vi "综合生物毒性电源命令.vi"(10 "通电/断电":bool, 11 "队列":refnum<queue>) -> (3 "队列输出":refnum<queue>)   [LabVIEW 2016, in "PLC.lvlib"]
uses:
  PLC.lvlib
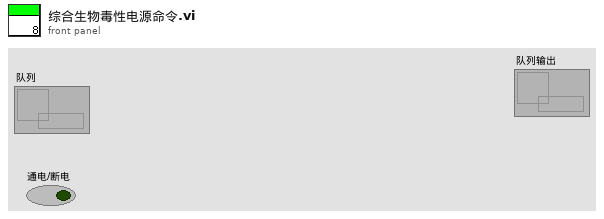
[diagram p1: front panel]
types:
  T1 = typedef "采配水类型.ctl" = enum16{"V1", "V2", "V3", "V4", "室内V1", "室内V2", "固定站V1", "固定站V2", "浮船V1", "浮船V2", "养殖尾水", "广东华南所"}
  T2 = cluster{"命令":string, "数据":cluster{"starting address":u16, "holding register value":u16}}
  T3 = cluster{"命令":string, "data":cluster{"starting address":u16, "coil values":bool[]}}
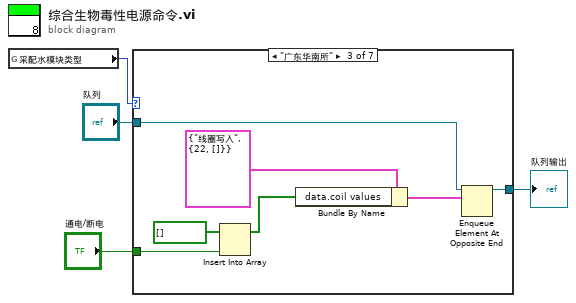
[diagram p0: block diagram]
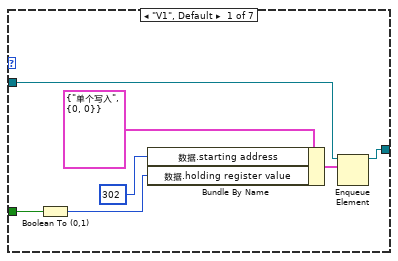
[diagram p2: hidden frame]
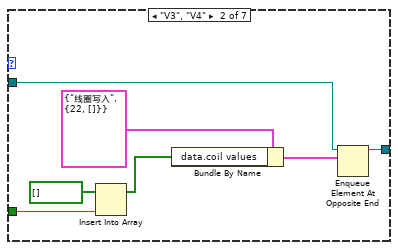
[diagram p3: hidden frame]
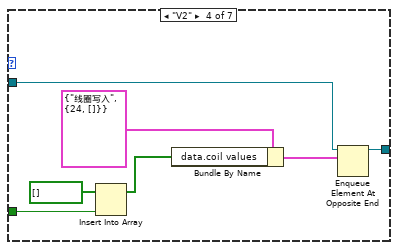
[diagram p4: hidden frame]
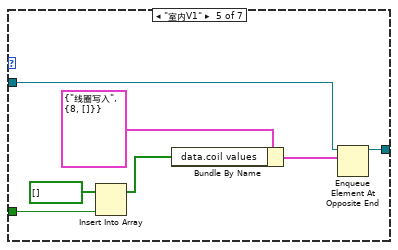
[diagram p5: hidden frame]
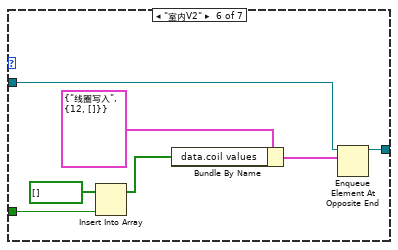
[diagram p6: hidden frame]
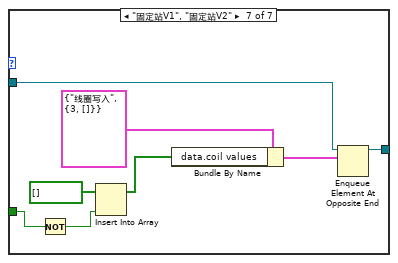
[diagram p7: hidden frame]
diagram:
  n1 = global read "系统设置全局变量.vi" "采配水模块类型"() -> (w1:T1)
  n2 = case shown="\"广东华南所\"" w1 {
    tunnel: "队列" -> [w9 w17 w24 w31 w38 w45 w53]
    tunnel: [w8 w16 w23 w30 w37 w44 w52] -> w3
    tunnel: "通电/断电" -> [w6 w15 w22 w29 w36 w43 w51]
    frame "V1", Default {
      n3 = Boolean To (0,1)(Boolean=w6) -> (0, 1=w5:i16)
      n4 = Bundle By Name(cluster=T2 {"命令"="单个写入", "数据"={"starting address"=0, "holding register value"=0}} ("元素"), "数据.starting address"=u16 302, "数据.holding register value"=w5) -> (w7:T2)
      n5 = Enqueue Element(queue=w9, element=w7) -> (queue out=w8:refnum<queue>)  [unwired: 2 in, 2 out]
    }
    frame "V3", "V4" {
      n6 = Insert Into Array(array=bool[] [] ("data.coil values"), new element=w15) -> (w12:bool[])  [unwired: 1 in]
      n7 = Bundle By Name(cluster=T3 {"命令"="线圈写入", "data"={"starting address"=22, "coil values"=[]}} ("元素"), "data.coil values"=w12) -> (w18:T3)
      n8 = Enqueue Element At Opposite End(queue=w17, element=w18) -> (queue out=w16:refnum<queue>)  [unwired: 2 in, 2 out]
    }
    frame "广东华南所" {
      n9 = Insert Into Array(array=bool[] [] ("data.coil values"), new element=w22) -> (w19:bool[])  [unwired: 1 in]
      n10 = Bundle By Name(cluster=T3 {"命令"="线圈写入", "data"={"starting address"=22, "coil values"=[]}} ("元素"), "data.coil values"=w19) -> (w25:T3)
      n11 = Enqueue Element At Opposite End(queue=w24, element=w25) -> (queue out=w23:refnum<queue>)  [unwired: 2 in, 2 out]
    }
    frame "V2" {
      n12 = Insert Into Array(array=bool[] [] ("data.coil values"), new element=w29) -> (w26:bool[])  [unwired: 1 in]
      n13 = Bundle By Name(cluster=T3 {"命令"="线圈写入", "data"={"starting address"=24, "coil values"=[]}} ("元素"), "data.coil values"=w26) -> (w32:T3)
      n14 = Enqueue Element At Opposite End(queue=w31, element=w32) -> (queue out=w30:refnum<queue>)  [unwired: 2 in, 2 out]
    }
    frame "室内V1" {
      n15 = Insert Into Array(array=bool[] [] ("data.coil values"), new element=w36) -> (w33:bool[])  [unwired: 1 in]
      n16 = Bundle By Name(cluster=T3 {"命令"="线圈写入", "data"={"starting address"=8, "coil values"=[]}} ("元素"), "data.coil values"=w33) -> (w39:T3)
      n17 = Enqueue Element At Opposite End(queue=w38, element=w39) -> (queue out=w37:refnum<queue>)  [unwired: 2 in, 2 out]
    }
    frame "室内V2" {
      n18 = Insert Into Array(array=bool[] [] ("data.coil values"), new element=w43) -> (w40:bool[])  [unwired: 1 in]
      n19 = Bundle By Name(cluster=T3 {"命令"="线圈写入", "data"={"starting address"=12, "coil values"=[]}} ("元素"), "data.coil values"=w40) -> (w46:T3)
      n20 = Enqueue Element At Opposite End(queue=w45, element=w46) -> (queue out=w44:refnum<queue>)  [unwired: 2 in, 2 out]
    }
    frame "固定站V1", "固定站V2" {
      n21 = Not(x=w51) -> (.not. x?=w47:bool)
      n22 = Insert Into Array(array=bool[] [] ("data.coil values"), new element=w47) -> (w48:bool[])  [unwired: 1 in]
      n23 = Bundle By Name(cluster=T3 {"命令"="线圈写入", "data"={"starting address"=3, "coil values"=[]}} ("元素"), "data.coil values"=w48) -> (w54:T3)
      n24 = Enqueue Element At Opposite End(queue=w53, element=w54) -> (queue out=w52:refnum<queue>)  [unwired: 2 in, 2 out]
    }
  }
  "队列输出" <- w3
